vi "CreateHTML.vi"(0 "reference in":refnum<class "Select.lvclass">, 2 "VI Name":string, 5 "error in (no error)":errorcluster) -> (13 "script dependencies":string[](array[string]), 14 "reference out":refnum<class "Select.lvclass">, 15 "HTML":string, 16 "js variables":string, 17 "js code for controls":string, 18 "js code for indicators":string, 19 "error out":errorcluster)   [LabVIEW 2014, in "FrontPanelPublisher.lvlib" / "Select.lvclass"]
uses:
  Select.lvclass
  Object_class/Object.lvclass
  Control_class/Control.lvclass
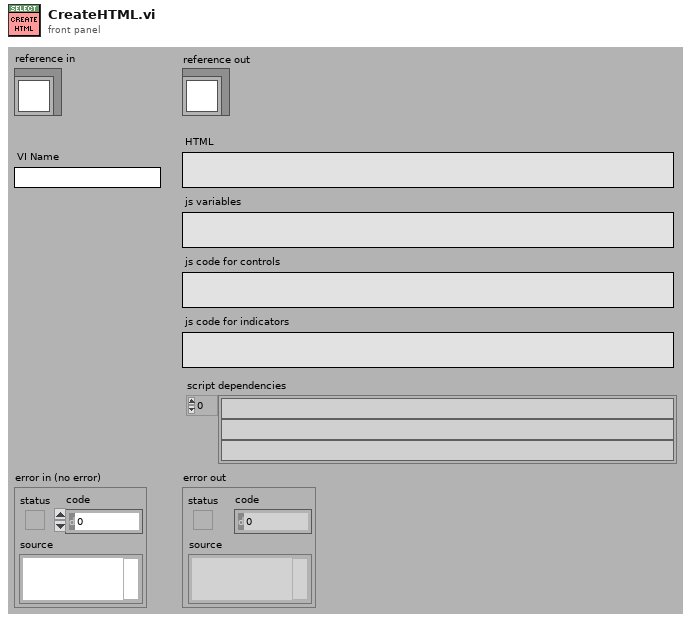
[diagram p1: front panel]
types:
  T1 = typedef "FrontPanelPublisher.lvlib/Object.lvclass/Attributes.ctl" = cluster{"UID":i32, "Type":string, "Coordinates":T2, "Reference":refnum<vi>}
  T2 = typedef "FrontPanelPublisher.lvlib/Object.lvclass/Coordinates.ctl" = cluster{"Left":i32, "Top":i32, "Height":u32, "Width":u32}
  T3 = typedef "FrontPanelPublisher.lvlib/Control.lvclass/Attributes.ctl" = cluster{"Description":string, "Indicator":bool, "Default Value":variant, "Control Index":i32, "Label":refnum<class "Text.lvclass">, "Caption":refnum<class "Text.lvclass">, "Use Picture":bool, "Image1 b64":string, "Image2 b64":string}
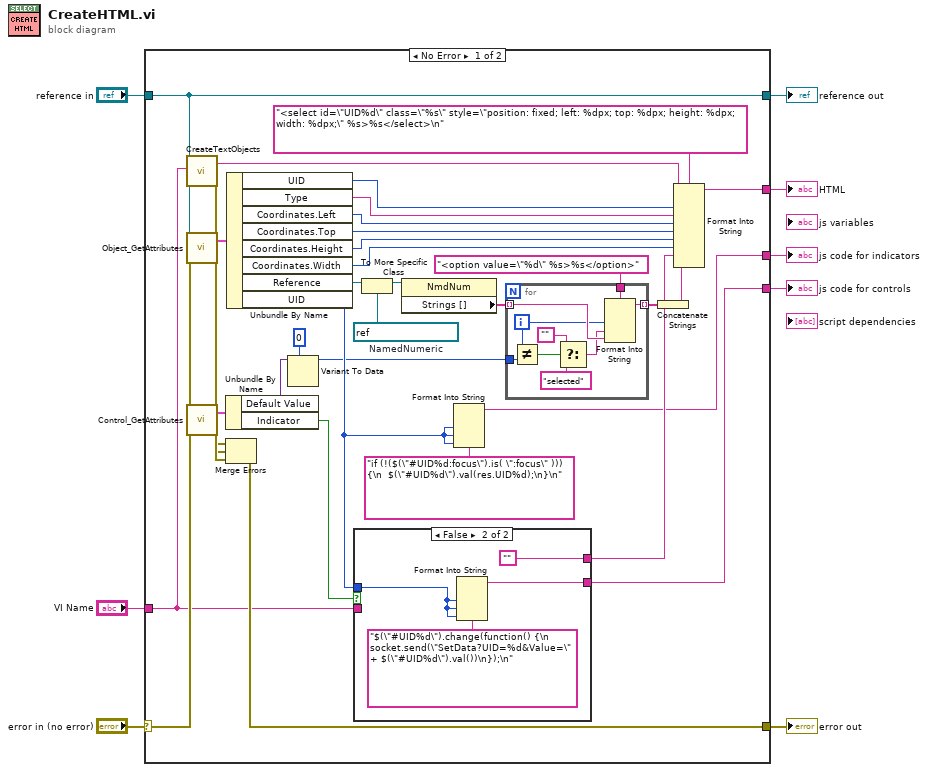
[diagram p0: block diagram]
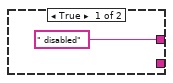
[diagram p2: hidden frame]
diagram:
  n1 = case shown="No Error" "error in (no error)" {
    selector: "error in (no error)" -> [w42 w58]
    tunnel: [w38 w58] -> w7
    tunnel: [w22 w57] -> w5
    tunnel: "reference in" -> [w22 w57]
    tunnel: [w32 _] -> w4
    tunnel: [w25 _] -> w3
    tunnel: [w27 _] -> w2
    tunnel: "VI Name" -> [w21 _]
    frame No Error {
      w18 = refnum<vi> refnum  # NamedNumeric
      n2 = call-dynamic "CreateTextObjects.vi"("reference in"=w22, "VI Name"=w21) -> ("HTML"=w23:string, "error out"=w39:errorcluster)  [unwired: 15 in, 1 out]
      n3 = call "Object_GetAttributes.vi"("reference in"=w22, "error in (no error)"=w42) -> ("Data"=w31:T1, "error out"=w40:errorcluster)  [unwired: 14 in, 2 out]
      n4 = call "Control_GetAttributes.vi"("reference in"=w22, "error in (no error)"=w42) -> ("Data"=w30:T3, "error out"=w41:errorcluster)  [unwired: 14 in, 2 out]
      n5 = Unbundle By Name(w30) -> ("Default Value"=w15:variant, "Indicator"=w29:bool)
      n6 = Merge Errors(w39, w40, w41) -> (w38:errorcluster)
      n7 = Unbundle By Name(w31) -> ("UID"=w36:i32, "Type"=w35:string, "Coordinates.Left"=w34:i32, "Coordinates.Top"=w33:i32, "Coordinates.Height"=w10:u32, "Coordinates.Width"=w9:u32, "Reference"=w20:refnum<vi>, "UID"=w24:i32)
      n8 = Variant To Data(type=0, Variant=w15) -> (data=w13:i32)  [unwired: 1 in, 1 out]
      n9 = case shown="False" w29 {
        tunnel: [" disabled" ""] -> w28
        tunnel: w24 -> [_ w54]
        tunnel: w21 -> [_ _]
        tunnel: [_ w53] -> w27
        frame True {
        }
        frame False {
          n10 = Format Into String(format string="$(\"#UID%d\").change(function() {\n  socket.send(\"SetData?UID=%d&Value=\" + $(\"#UID%d\").val())\n});\n", w54, w54, w54) -> (resulting string=w53:string)  [unwired: 2 in, 1 out]
        }
      }
      n11 = To More Specific Class(target class=w18, reference=w20) -> (specific class reference=w19:refnum<vi>)  [unwired: 1 in, 1 out]
      n12 = property class="NmdNum"(reference=w19) -> ("Strings []"=w17:string[])  [unwired: 1 in, 2 out]
      n13 = Format Into String(format string="if (!($(\"#UID%d:focus\").is( \":focus\" ))) {\n  $(\"#UID%d\").val(res.UID%d);\n}\n", w24, w24, w24) -> (resulting string=w25:string)  [unwired: 2 in, 1 out]
      n14 = for {
        tunnel: w17 -> [w50] mode=indexing
        tunnel: "<option value=\"%d\" %s>%s</option>" -> [w51]
        tunnel: w13 -> [w48]
        tunnel: [w46] -> w12 mode=indexing
        i -> [w45]
        n15 = Not Equal?(x=w45, y=w48) -> (x != y?=w49:bool)
        n16 = Select(t="", s=w49, f="selected") -> (s? t:f=w47:string)
        n17 = Format Into String(format string=w51, w45, w47, w50) -> (resulting string=w46:string)  [unwired: 2 in, 1 out]
      }
      n18 = Concatenate Strings(w12) -> (w11:string)
      n19 = Format Into String(format string="<select id=\"UID%d\" class=\"%s\" style=\"position: fixed; left: %dpx; top: %dpx; height: %dpx; width: %dpx;\" %s>%s</select>\n", initial string=w23, w36, w35, w34, w33, w10, w9, w28, w11) -> (resulting string=w32:string)  [unwired: 1 in, 1 out]
    }
    frame Error {
    }
  }
  "error out" <- w7
  "reference out" <- w5
  "HTML" <- w4
  "js code for controls" <- w2
  "js code for indicators" <- w3
